vi "SetParam.vi"(8 "error in (no error)":errorcluster caption="entrée d'erreur (pas d'erreur)", 10 "LeavePOut":cluster{"p":i32}={"p"=2}, 11 "LeavePOut.lvclass":refnum<class "LeavePOut.lvclass">) -> (0 "error out":errorcluster caption="sortie d'erreur", 3 "LeavePOut.lvclass":refnum<class "LeavePOut.lvclass">)   [LabVIEW 2020, in "LeavePOut.lvclass"]
doc: "Set Parameters"
uses:
  LeavePOut.lvclass
  LeavePOut.lvclass/LeavePOut.ctl
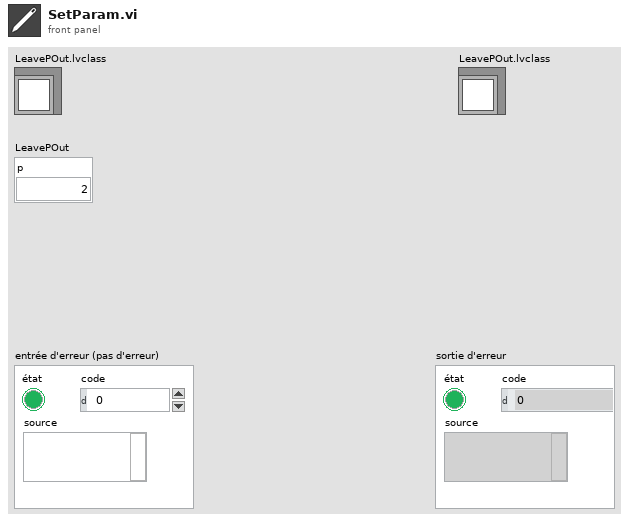
[diagram p1: front panel]
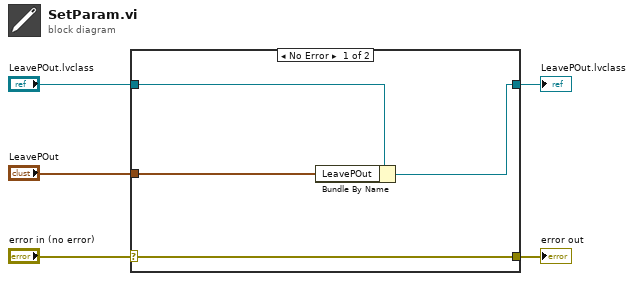
[diagram p0: block diagram]
diagram:
  n1 = case shown="No Error" "error in (no error)" {
    selector: "error in (no error)" -> [w9 w10]
    tunnel: [w9 w10] -> w4
    tunnel: [w7 w11] -> w2
    tunnel: "LeavePOut.lvclass" -> [w8 w11]
    tunnel: "LeavePOut" -> [w6 _]
    frame No Error {
      n2 = Bundle By Name(cluster=w8, "LeavePOut"=w6) -> (w7:refnum<class "LeavePOut.lvclass">)
    }
    frame Error {
    }
  }
  "error out" <- w4
  "LeavePOut.lvclass" <- w2
